vi "write_attributes.vi"(8 "error in (no error)":errorcluster, 10 "attributes":T1, 11 "OPTICS in":refnum<class "OPTICS.lvclass">) -> (0 "error out":errorcluster, 3 "OPTICS out":refnum<class "OPTICS.lvclass">)   [LabVIEW 2020, in "OPTICS.lvclass"]
uses:
  OPTICS.lvclass
  Controls/optics_attributes.ctl
  OPTICS.lvclass/OPTICS.ctl
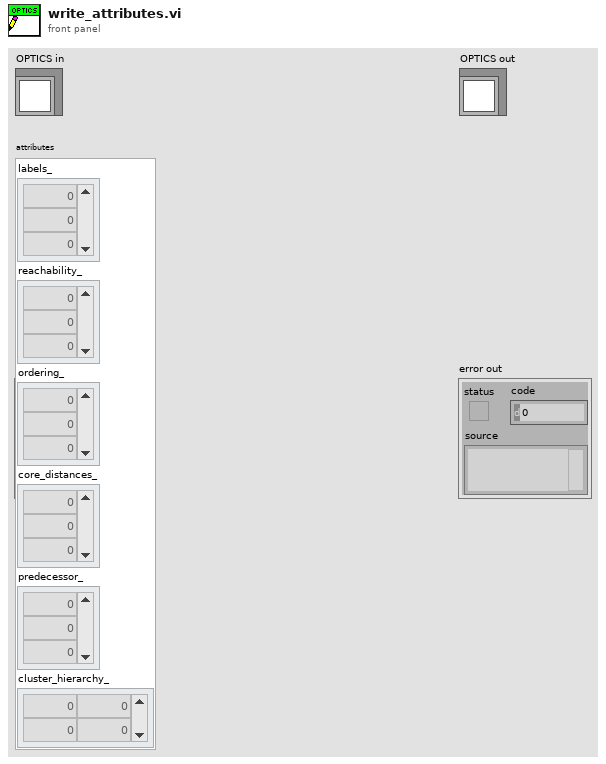
[diagram p1: front panel]
types:
  T1 = typedef "optics_attributes.ctl" = cluster{"labels_":dbl[], "reachability_":dbl[], "ordering_":dbl[], "core_distances_":dbl[], "predecessor_":dbl[], "cluster_hierarchy_":dbl[][]}
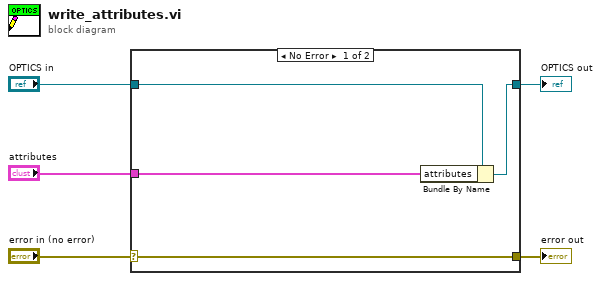
[diagram p0: block diagram]
diagram:
  n1 = case shown="No Error" "error in (no error)" {
    selector: "error in (no error)" -> [w9 w10]
    tunnel: [w9 w10] -> w4
    tunnel: [w7 w11] -> w2
    tunnel: "OPTICS in" -> [w8 w11]
    tunnel: "attributes" -> [w6 _]
    frame No Error {
      n2 = Bundle By Name(cluster=w8, "attributes"=w6) -> (w7:refnum<class "OPTICS.lvclass">)
    }
    frame Error {
    }
  }
  "error out" <- w4
  "OPTICS out" <- w2
